vi "FPGA image acquisition.vi"   [LabVIEW 2012]
uses:
  <vilib>/eio/EIONode/EIONode.xnode
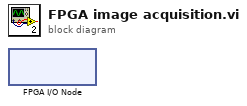
[diagram p0: block diagram]
diagram:
  n1 = xnode "FPGA I/O Node"() -> ()  [unwired: 1 in, 2 out]
